vi "Generate Channels Dialog.vi"() -> (1 "Cancel Out":bool, 2 "allowed classifications":T1[](array[typedef])=[enum."output data"])   [LabVIEW 2014, in "Scan Engine editor node.lvclass"]
uses:
  Scan Engine editor node.lvclass
  <vilib>/NI/Tag Bus Module Framework/channel/channel classification.ctl
  <vilib>/NI/Tag Bus Module Framework/channel/TBM channel.lvclass
panel:
  in  "Cancel":bool
  in  "OK":bool
  in  "Tags":enum32{"M2E", "E2M", "ALL"}(radio)
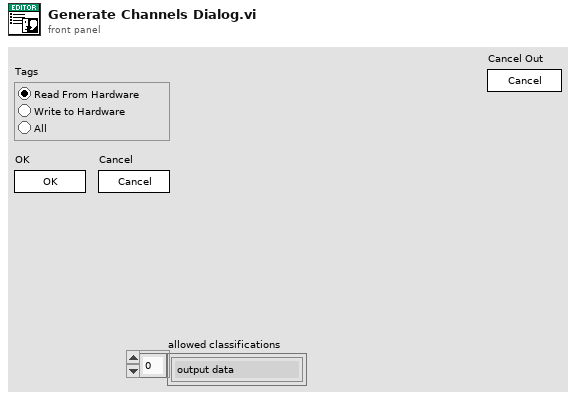
[diagram p1: front panel]
types:
  T1 = typedef "TBM channel.lvclass/channel classification.ctl" = enum16{"input data", "output data", "processing parameter", "processing result"}
  T2 = enum32{"Invalid", "Standard", "Closed", "Hidden", "Minimized", "Maximized"}
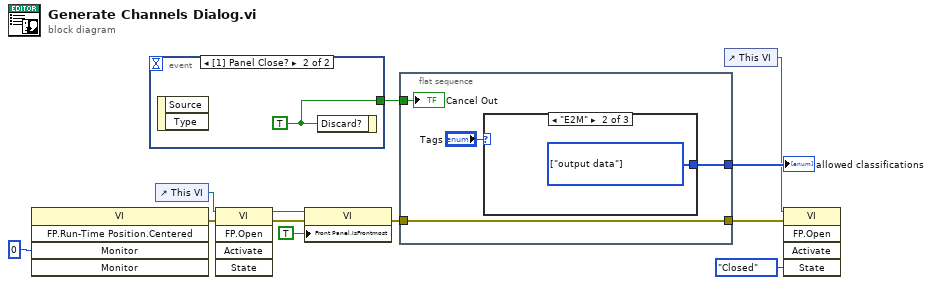
[diagram p0: block diagram]
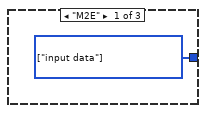
[diagram p2: hidden frame]
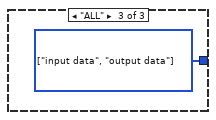
[diagram p3: hidden frame]
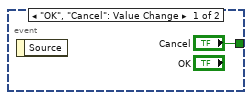
[diagram p4: hidden frame]
diagram:
  n1 = invoke class="VI" method="FP.Run-Time Position.Centered"("Monitor"=i16 0) -> (error out=w2:errorcluster)  [unwired: 4 in, 4 out]
  n2 = event shown="[1] Panel Close?" {
    selector: _ -> [_ _]
    dyn-events: _ -> [_ _]
    timeout: _ -> [_ _]
    tunnel: ["Cancel" w14] -> w12
    event "OK", "Cancel": Value Change {
      n3 = event-data() -> ()  [unwired: 1 in, 1 out]
    }
    event Panel Close? {
      w14 = TRUE ("Discard?")
      n4 = event-data() -> ()  [unwired: 1 in, 2 out]
      n5 = event-data("Discard?"=w14) -> ()  [unwired: 1 in, 1 out]
    }
  }
  n6 = control-ref of="This VI"() -> (w10:refnum<vi>)
  n7 = invoke class="VI" method="FP.Open"(reference=w10, error in=w2) -> (reference out=w9:refnum<vi>, error out=w8:errorcluster)  [unwired: 3 in, 3 out]
  n8 = property class="VI"(reference=w9, error in=w8, "Front Panel.IsFrontmost"=TRUE ("Front Panel Window:Is Frontmost")) -> (error out=w1:errorcluster)  [unwired: 1 out]
  n9 = flat-sequence {
    tunnel: w12 -> [w18]
    tunnel: [w16] -> w11
    tunnel: w1 -> [w15]
    tunnel: [w15] -> w4
    frame #0 {
      n10 = case shown="\"E2M\"" "Tags" {
        tunnel: [w19 w20 w21] -> w16
        frame "M2E" {
          w19 = T1[] [enum."input data"] items=["input data", "output data", "processing parameter", "processing result"] ("allowed classifications")
        }
        frame "E2M" {
          w20 = T1[] [enum."output data"] items=["input data", "output data", "processing parameter", "processing result"] ("allowed classifications")
        }
        frame "ALL" {
          w21 = T1[] [enum."input data", enum."output data"] items=["input data", "output data", "processing parameter", "processing result"] ("allowed classifications")
        }
      }
      "Cancel Out" <- w18
    }
  }
  n11 = control-ref of="This VI"() -> (w5:refnum<vi>)
  n12 = invoke class="VI" method="FP.Open"(reference=w5, error in=w4, "State"=T2."Closed") -> ()  [unwired: 2 in, 5 out]
  "allowed classifications" <- w11
